vi "Equip-Set active (string).vi"(0 "Config Name":string, 11 "error in (no error)":errorcluster) -> (15 "error out":errorcluster)   [LabVIEW 2020]
uses:
  <vilib>/Utility/config.llb/Write Key (String).vi
  <vilib>/Utility/config.llb/NI_LVConfig.lvlib
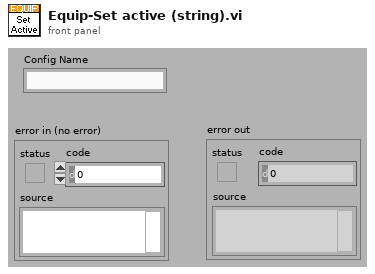
[diagram p1: front panel]
types:
  T1 = typedef "NI_LVConfig.lvlib/Config Data RefNum.ctl" = refnum<k1>
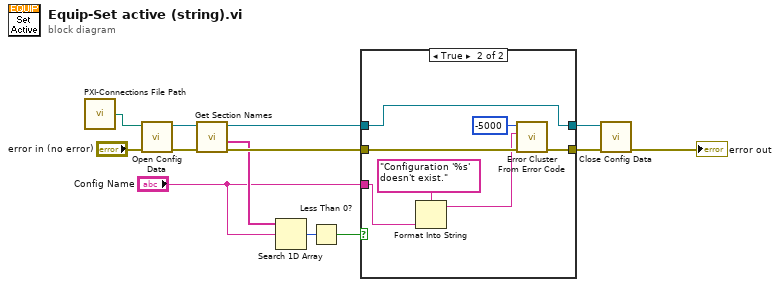
[diagram p0: block diagram]
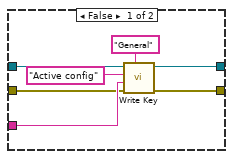
[diagram p2: hidden frame]
diagram:
  n1 = call "PXI-Connections File Path.vi"() -> ("Path"=w1:path)  [unwired: 1 in]
  n2 = call <vilib>:"Open Config Data.vi"("error in (no error)"="error in (no error)", "configuration file path"=w1) -> ("error out"=w12:errorcluster, "refnum"=w11:T1)  [unwired: 7 in, 1 out]
  n3 = call <vilib>:"Get Section Names.vi"("error in (no error)"=w12, "refnum"=w11) -> ("error out"=w10:errorcluster, "section names"=w5:string[], "refnum out"=w9:T1)  [unwired: 7 in]
  n4 = Search 1D Array(1D array=w5, element="Config Name") -> (index of element=w3:i32)  [unwired: 1 in]
  n5 = Less Than 0?(x=w3) -> (x < 0?=w8:bool)
  n6 = case shown="True" w8 {
    tunnel: [w15 w27] -> w7
    tunnel: "Config Name" -> [w19 w24]
    tunnel: w10 -> [w18 w26]
    tunnel: w9 -> [w17 w21]
    tunnel: [w14 w21] -> w6
    frame False {
      n7 = call-poly <vilib>:"Write Key.vi"("section"="General", "error in (no error)"=w18, "value"=w19, "key"="Active config", "refnum"=w17) -> ("error out"=w15:errorcluster, "refnum out"=w14:T1)  [unwired: 4 in, 1 out]
    }
    frame True {
      n8 = Format Into String(format string="Configuration '%s' doesn't exist.", w24) -> (resulting string=w23:string)  [unwired: 2 in, 1 out]
      n9 = call <vilib>:"Error Cluster From Error Code.vi"("error in (no error)"=w26, "error message (\"\")"=w23, "error code (0)"=-5000) -> ("error out"=w27:errorcluster)  [unwired: 6 in]
    }
  }
  n10 = call <vilib>:"Close Config Data.vi"("error in (no error)"=w7, "refnum"=w6) -> ("error out"=→"error out":errorcluster)  [unwired: 8 in, 1 out]
